vi "Skip.vi"(7 "Description":string, 8 "error in (no error)":errorcluster, 9 "Message":string, 11 "LUnit Test Case In":refnum<class "LUnit Test Case V2.lvclass">) -> (0 "error out":errorcluster, 3 "LUnit Test Case Out":refnum<class "LUnit Test Case V2.lvclass">)   [LabVIEW 2020, in "LUnit Test Case V2.lvclass"]
doc: "Ignores results from the calling test method when evaluating the test case result. A description and message may be provided."
uses:
  LUnit Test Case V2.lvclass
  Result/Result.ctl
  Result/Status.ctl
  Result/Type.ctl
  LUnit Test Case V2.lvclass/LUnit Test Case V2.ctl
  Result/Result.lvlib
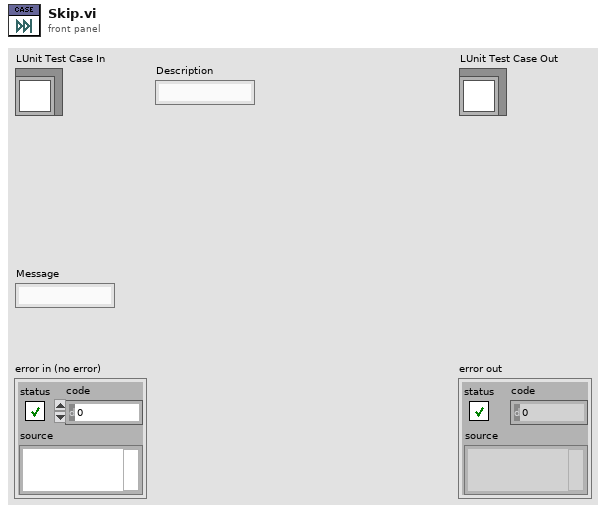
[diagram p1: front panel]
types:
  T1 = typedef "Result.lvlib/Result.ctl" = cluster{"Case":string, "Method":string, "Message":string, "Description":string, "Status":T2, "Result Type":T3}
  T2 = typedef "Result.lvlib/Status.ctl" = enum16{"Pass", "Fail", "Error", "Skipped", "Setup Error", "Broken", "Teardown Error"}
  T3 = typedef "Result.lvlib/Type.ctl" = enum16{"None", "Pass", "Fail", "Skip", "Pass if Equal", "Fail if Equal", "Pass if Error", "Fail if Error", "Pass if", "Fail if"}
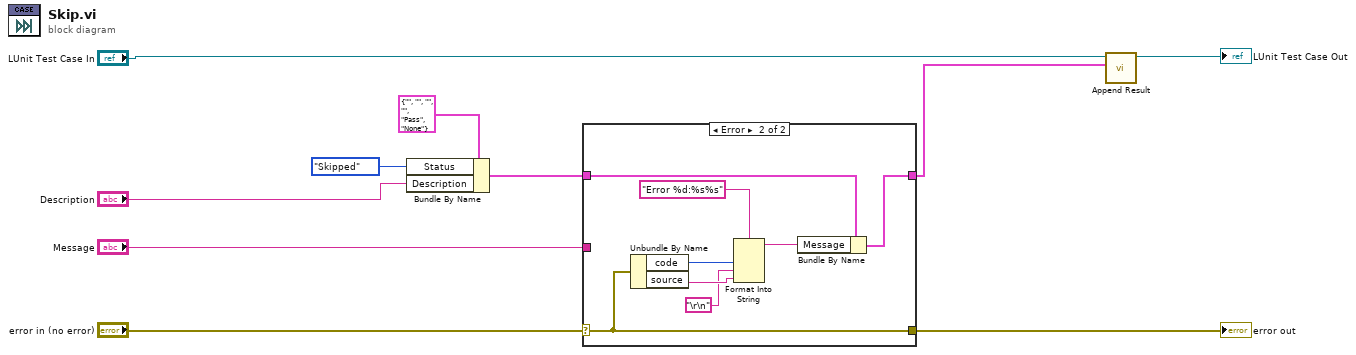
[diagram p0: block diagram]
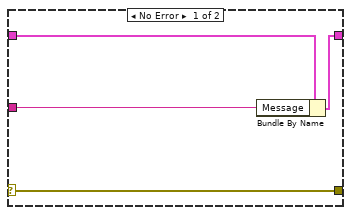
[diagram p2: hidden frame]
diagram:
  n1 = Bundle By Name(cluster=T1 {"Case"="", "Method"="", "Message"="", "Description"="", "Status"=enum."Pass", "Result Type"=enum."None"} ("Temporary Assertion Result"), "Status"=Status."Skipped", "Description"="Description") -> (w4:T1)
  n2 = case shown="Error" "error in (no error)" {
    selector: "error in (no error)" -> [w14 w21]
    tunnel: [w14 w21] -> w9
    tunnel: [w12 w22] -> w1
    tunnel: "Message" -> [w13 _]
    tunnel: w4 -> [w11 w15]
    frame No Error {
      n3 = Bundle By Name(cluster=w11, "Message"=w13) -> (w12:T1)
    }
    frame Error {
      n4 = Unbundle By Name(w21) -> ("code"=w19:i32, "source"=w17:string)
      n5 = Format Into String(format string="Error %d:%s%s", w19, "\r\n", w17) -> (resulting string=w18:string)  [unwired: 2 in, 1 out]
      n6 = Bundle By Name(cluster=w15, "Message"=w18) -> (w22:T1)
    }
  }
  "error out" <- w9
  n7 = call "Append Result.vi"("Result"=w1, "LUnit Test Case V2 in"="LUnit Test Case In") -> ("LUnit Test Case V2 out"=→"LUnit Test Case Out":refnum<class "LUnit Test Case V2.lvclass">)  [unwired: 9 in]
